vi "Configure Step Detection.vi"(8 "error in (no error)":errorcluster, 10 "Step Det":bool, 11 "RS Z2X in":refnum<class "RS Z2X.lvclass">) -> (0 "error out":errorcluster, 3 "RS Z2X out":refnum<class "RS Z2X.lvclass">)   [LabVIEW 2020, in "RS Z2X.lvclass"]
uses:
  RS Z2X.lvclass
  Power Meter.lvclass
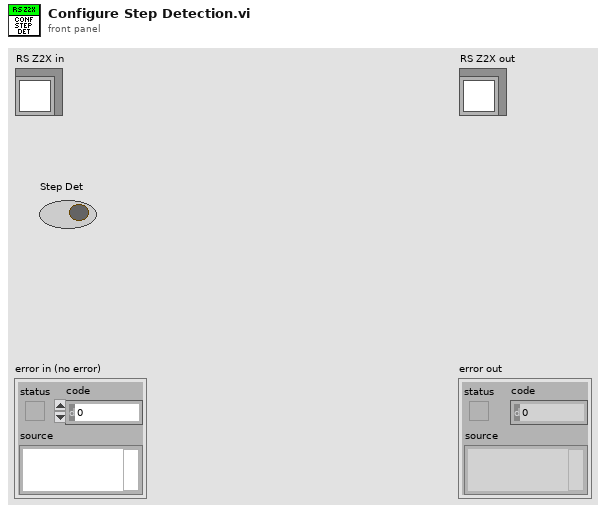
[diagram p1: front panel]
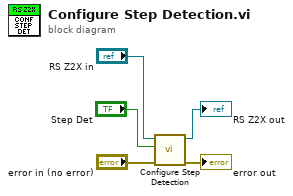
[diagram p0: block diagram]
diagram:
  n1 = call-parent "Configure Step Detection.vi"("error in (no error)"="error in (no error)", "Step Det"="Step Det", "Power Meter in"="RS Z2X in") -> ("error out"=→"error out":errorcluster, "Power Meter out"=→"RS Z2X out":refnum<class "RS Z2X.lvclass">)  [unwired: 7 in]
